vi "AMCS_Glbl_test.vi"() -> ()   [LabVIEW 2012]
uses:
  AMCS_Data.vi
panel:
  out "AMCS_Profile":i32
  out "Raw Uncorrected Return":u16[][](graph)
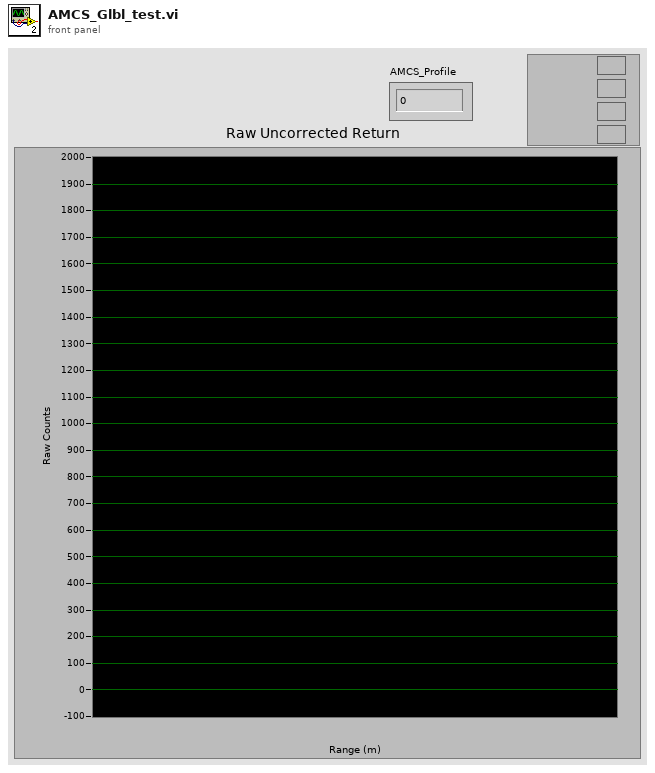
[diagram p1: front panel]
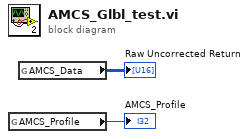
[diagram p0: block diagram]
diagram:
  n1 = global read "AMCS_Data.vi" "AMCS_Profile"() -> (→"AMCS_Profile":i32)
  n2 = global read "AMCS_Data.vi" "AMCS_Data"() -> (→"Raw Uncorrected Return":u16[][])
